vi "Overlay crosshairs.vi"(0 "Refnum in":T1, 1 "X Resolution":i32, 2 "Y Resolution":i32, 5 "centerline crosshair":T2={"position"=160.0, "color"=16769536, "width"=0.0}, 7 "horizontal crosshair HIGH":T2={"position"=56.0, "color"=16711680, "width"=0.0}, 9 "horizontal crosshair LO":T2={"position"=100.0, "color"=255, "width"=0.0}, 11 "error in (no error)":errorcluster) -> (4 "Refnum out":T1, 15 "error out":errorcluster)   [LabVIEW 2020]
uses:
  <vilib>/vision/Image Controls.llb/IMAQ Image.ctl
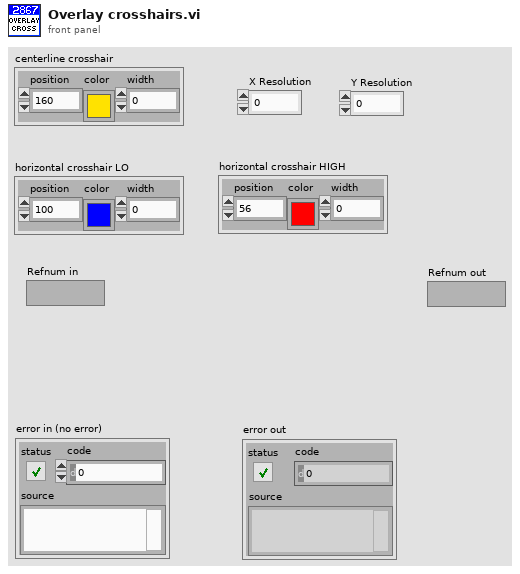
[diagram p1: front panel]
types:
  T1 = typedef "IMAQ Image.ctl" = refnum<image>
  T2 = cluster{"position":dbl, "color":u32, "width":dbl}
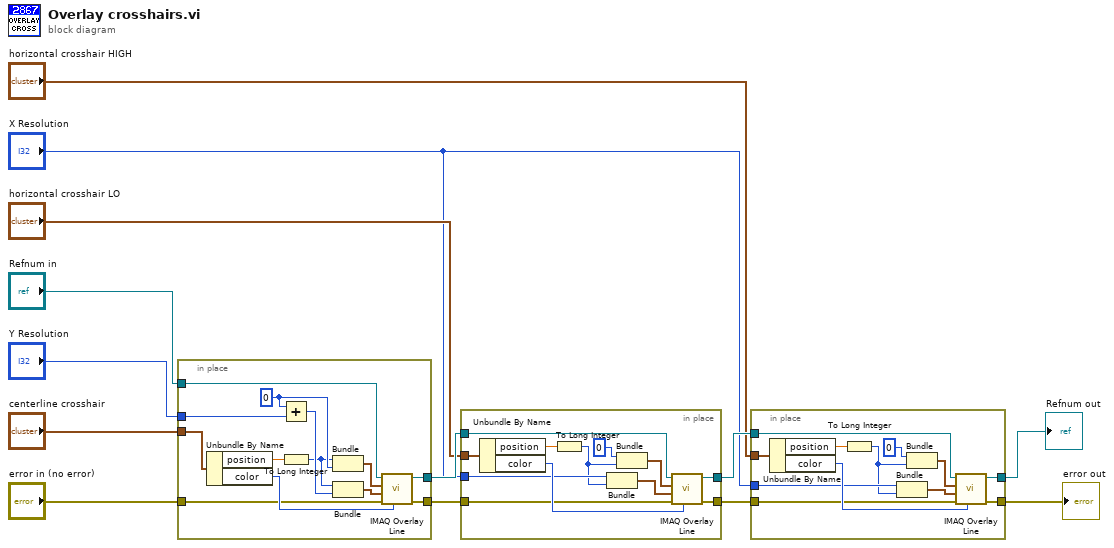
[diagram p0: block diagram]
diagram:
  n1 = in-place {
    in-place-border: [w15] -> w10
    in-place-border: "Refnum in" -> [w25]
    in-place-border: "Y Resolution" -> [w20]
    in-place-border: "centerline crosshair" -> [w17]
    in-place-border: "error in (no error)" -> [w16]
    in-place-border: [w14] -> w8
    w22 = 0
    n2 = Unbundle By Name(w17) -> ("position"=w19:dbl, "color"=w26:u32)
    n3 = Add(x=w22, y=w20) -> (x+y=w21:i32)
    n4 = To Long Integer(number=w19) -> (32bit integer=w18:i32)
    n5 = Bundle(w18, w22) -> (w24:cluster{i32, i32})  [unwired: 1 in]
    n6 = Bundle(w18, w21) -> (w23:cluster{i32, i32})  [unwired: 1 in]
    n7 = call "IMAQ Overlay Line"("Color"=w26, "error in (no error)"=w16, "End Point"=w23, "Start Point"=w24, "Image"=w25) -> ("error out"=w14:errorcluster, "Image Out"=w15:T1)  [unwired: 5 in]
  }
  n8 = in-place {
    in-place-border: [w38] -> w7
    in-place-border: w10 -> [w36]
    in-place-border: "horizontal crosshair LO" -> [w32]
    in-place-border: w8 -> [w31]
    in-place-border: "X Resolution" -> [w29]
    in-place-border: [w28] -> w6
    n9 = Unbundle By Name(w32) -> ("position"=w33:dbl, "color"=w37:u32)
    n10 = To Long Integer(number=w33) -> (32bit integer=w27:i32)
    n11 = Bundle("X Resolution"=w29, w27) -> (w34:cluster{"X Resolution":i32, i32})  [unwired: 1 in]
    n12 = Bundle(0, w27) -> (w35:cluster{i32, i32})  [unwired: 1 in]
    n13 = call "IMAQ Overlay Line"("Color"=w37, "error in (no error)"=w31, "End Point"=w34, "Start Point"=w35, "Image"=w36) -> ("error out"=w28:errorcluster, "Image Out"=w38:T1)  [unwired: 5 in]
  }
  n14 = in-place {
    in-place-border: [w50] -> w2
    in-place-border: w7 -> [w48]
    in-place-border: "horizontal crosshair HIGH" -> [w44]
    in-place-border: w6 -> [w43]
    in-place-border: "X Resolution" -> [w41]
    in-place-border: [w40] -> w3
    n15 = Unbundle By Name(w44) -> ("position"=w45:dbl, "color"=w49:u32)
    n16 = To Long Integer(number=w45) -> (32bit integer=w39:i32)
    n17 = Bundle("X Resolution"=w41, w39) -> (w46:cluster{"X Resolution":i32, i32})  [unwired: 1 in]
    n18 = Bundle(0, w39) -> (w47:cluster{i32, i32})  [unwired: 1 in]
    n19 = call "IMAQ Overlay Line"("Color"=w49, "error in (no error)"=w43, "End Point"=w46, "Start Point"=w47, "Image"=w48) -> ("error out"=w40:errorcluster, "Image Out"=w50:T1)  [unwired: 5 in]
  }
  "Refnum out" <- w2
  "error out" <- w3
